vi "DSF.Shared.Configuration.Framework.Set Cycle Timing Factors.vi"(8 "error in (no error)":errorcluster, 10 "Cycle Timing Factors":T1={"Decimation"=1, "Offset"=0}, 11 "Framework Configuration in":refnum<class "DSF.Shared.Configuration.Framework.lvclass">) -> (0 "error out":errorcluster, 3 "Framework Configuration out":refnum<class "DSF.Shared.Configuration.Framework.lvclass">)   [LabVIEW 2016, in "DSF.Shared.lvlib" / "DSF.Shared.Configuration.Framework.lvclass"]
uses:
  DSF.Shared.Configuration.Framework.lvclass
  Typedefs/DSF.Shared.Typedefs.Cycle Timing Factors.ctl
  DSF.Shared.Configuration.Framework.lvclass/DSF.Shared.Configuration.Framework.ctl
  DSF.Shared.lvlib
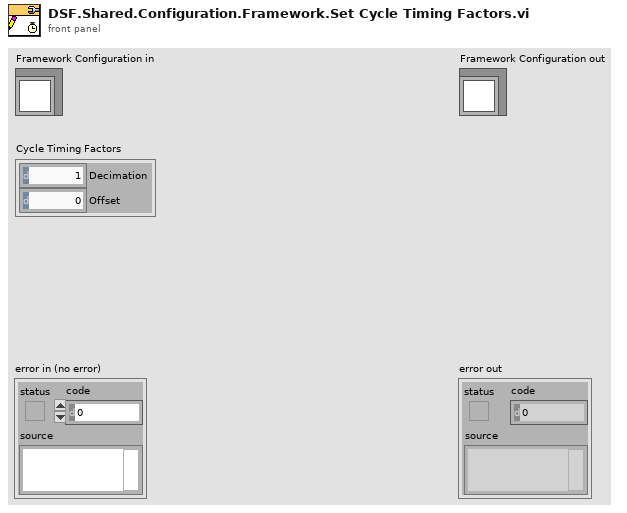
[diagram p1: front panel]
types:
  T1 = typedef "DSF.Shared.lvlib/DSF.Shared.Typedefs.Cycle Timing Factors.ctl" = cluster{"Decimation":u64, "Offset":u64}
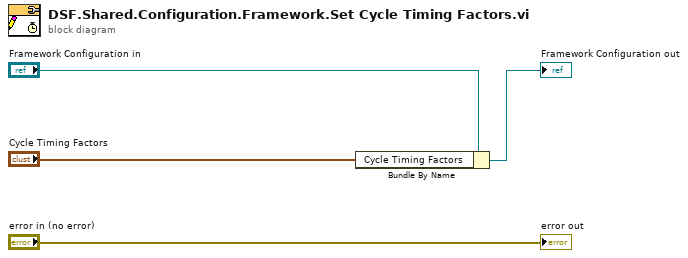
[diagram p0: block diagram]
diagram:
  n1 = Bundle By Name(cluster="Framework Configuration in", "Cycle Timing Factors"="Cycle Timing Factors") -> (→"Framework Configuration out":refnum<class "DSF.Shared.Configuration.Framework.lvclass">)
  "error out" <- "error in (no error)"
